vi "Mavlink CRC READ.vi"(11 "Byte IN":u8[](array[numeric])=[9, 19, 1, 1, 0, 0, 0, 0, 0, 2, 3, 81, 4, 3]) -> (3 "CRC":bool)   [LabVIEW 2023]
panel:
  out "Incoming Checksum":u16
  out "Calculated Checksum":u16
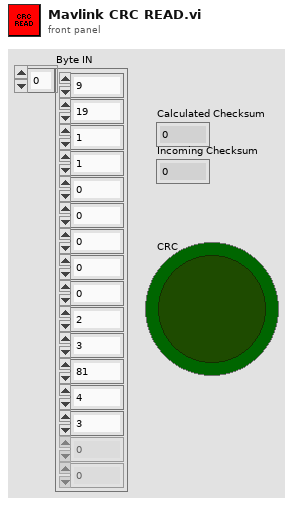
[diagram p1: front panel]
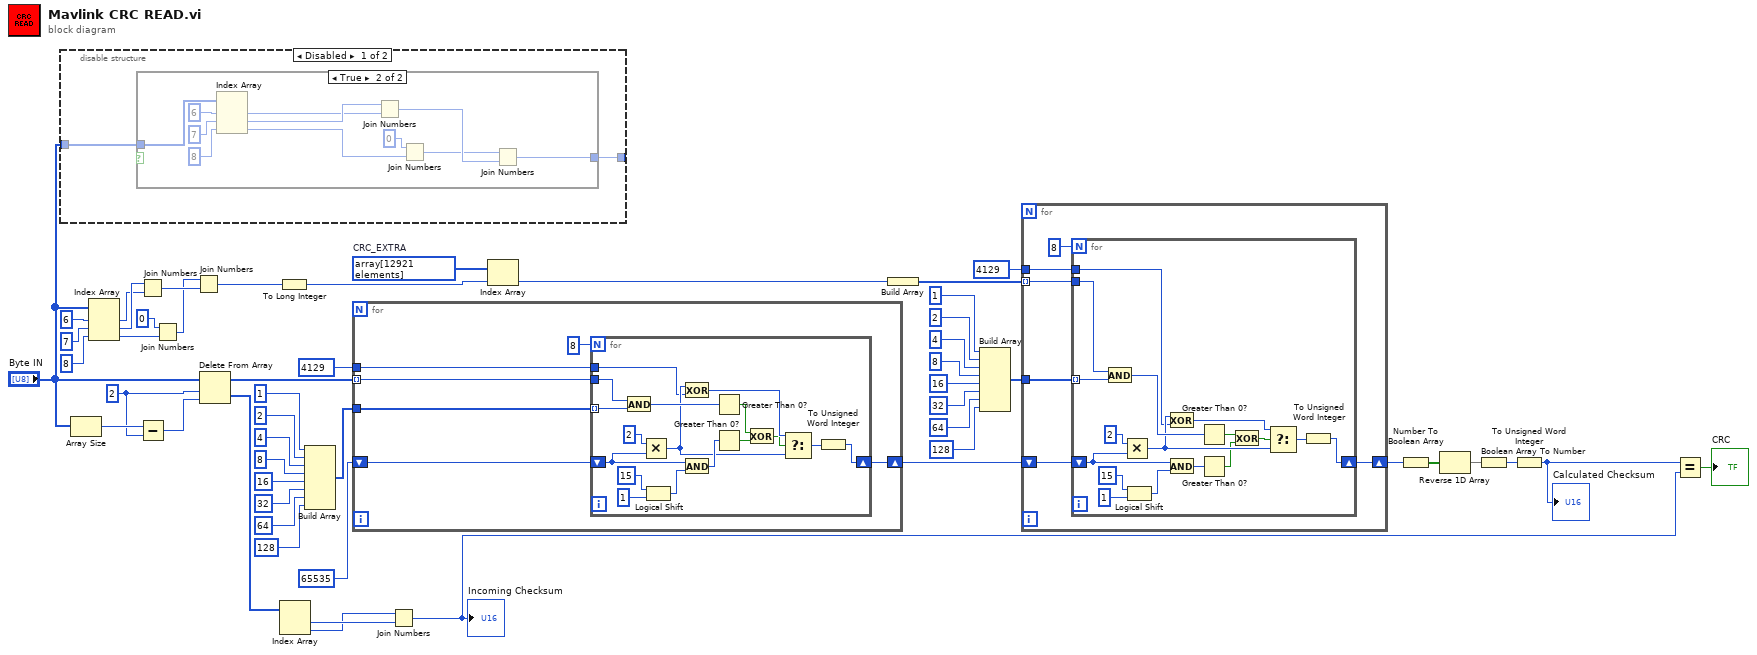
[diagram p0: block diagram]
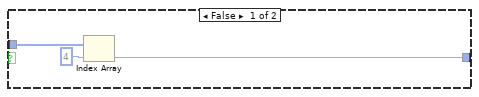
[diagram p2: hidden frame]
diagram:
  w20 = 2 ("y")
  w25 = u8[] array[12921 elements]  # CRC_EXTRA
  n1 = disable-structure shown="Disabled" {
    disable-tunnel: "Byte IN" -> [w53 _]
    disable-tunnel: [w52 _] -> _
    frame Disabled {
      n2 = case shown="True" {
        selector: _ -> [_ _]
        tunnel: w53 -> [w56 w57]
        tunnel: [w54 w58] -> w52
        frame False {
          n3 = Index Array(array=w56, index=4) -> (element=w54:u8)
        }
        frame True {
          n4 = Index Array(array=w57, index #1=6 ("index"), index #2=7 ("index"), index #3=8 ("index")) -> (element #1=w63:u8, element #2=w64:u8, element #3=w65:u8)
          n5 = Join Numbers(hi=w64, lo=w63) -> ((hi.lo)=w67:u16)
          n6 = Join Numbers(hi=u8 0, lo=w65) -> ((hi.lo)=w66:u16)
          n7 = Join Numbers(hi=w66, lo=w67) -> ((hi.lo)=w58:u32)
        }
      }
    }
    frame Enabled {
    }
  }
  n8 = Array Size(array="Byte IN") -> (size(s)=w22:i32)
  n9 = Index Array(array="Byte IN", index #1=6 ("index"), index #2=7 ("index"), index #3=8 ("index")) -> (element #1=w7:u8, element #2=w8:u8, element #3=w9:u8)
  n10 = Join Numbers(hi=w8, lo=w7) -> ((hi.lo)=w11:u16)
  n11 = Subtract(x=w22, y=w20) -> (x-y=w21:i32)
  n12 = Join Numbers(hi=u8 0, lo=w9) -> ((hi.lo)=w10:u16)
  n13 = Join Numbers(hi=w10, lo=w11) -> ((hi.lo)=w1:u32)
  n14 = Delete From Array(array="Byte IN", length=w20, index=w21) -> (deleted portion=w19:u8[], array with subset deleted=w18:u8[])
  n15 = To Long Integer(number=w1) -> (32bit integer=w12:i32)
  n16 = Index Array(array=w19) -> (element #1=w14:u8, element #2=w13:u8)  [unwired: 2 in]
  n17 = Build Array(u8 1, u8 2, u8 4, u8 8, u8 16, u8 32, u8 64, u8 128) -> (w42:u8[])
  n18 = for {
    shift-right: [w71] -> w26
    shift-left: u16 65535 -> [w73]
    tunnel: w18 -> [w70] mode=indexing
    tunnel: w42 -> [w69]
    tunnel: u16 4129 -> [w68]
    n19 = for {
      N: 8 -> [_]
      shift-right: [w89] -> w71
      shift-left: w73 -> [w79]
      tunnel: w69 -> [w80] mode=indexing
      tunnel: w70 -> [w75]
      tunnel: w68 -> [w74]
      n20 = And(x=w75, y=w80) -> (x .and. y?=w87:u8)
      n21 = Multiply(x=u16 2, y=w79) -> (x*y=w81:u16)
      n22 = Logical Shift(y=u16 15 ("Numeric"), x=u16 1 ("Numeric 2")) -> (x << y=w83:u16)
      n23 = Exclusive Or(1:w74, 2:w81) -> (0:w90:u16)
      n24 = And(x=w79, y=w83) -> (x .and. y?=w82:u16)
      n25 = Greater Than 0?(x=w87) -> (x > 0?=w86:bool)
      n26 = Greater Than 0?(x=w82) -> (x > 0?=w77:bool)
      n27 = Exclusive Or(1:w77, 2:w86) -> (0:w76:bool)
      n28 = Select(t=w90, s=w76, f=w81) -> (s? t:f=w88:u16)
      n29 = To Unsigned Word Integer(number=w88) -> (unsigned 16bit integer=w89:u16)
    }
  }
  n30 = Join Numbers(hi=w13, lo=w14) -> ((hi.lo)=w16:u16)
  "Incoming Checksum" <- w16
  n31 = Index Array(array=w25, index=w12) -> (element=w24:u8)
  n32 = Build Array(w24) -> (w23:u8[])
  n33 = Build Array(u8 1, u8 2, u8 4, u8 8, u8 16, u8 32, u8 64, u8 128) -> (w36:u8[])
  n34 = for {
    shift-right: [w94] -> w27
    shift-left: w26 -> [w96]
    tunnel: w36 -> [w93]
    tunnel: u16 4129 -> [w92]
    tunnel: w23 -> [w91] mode=indexing
    n35 = for {
      N: 8 -> [_]
      shift-right: [w112] -> w94
      shift-left: w96 -> [w102]
      tunnel: w93 -> [w103] mode=indexing
      tunnel: w91 -> [w98]
      tunnel: w92 -> [w97]
      n36 = And(x=w98, y=w103) -> (x .and. y?=w110:u8)
      n37 = Multiply(x=u16 2, y=w102) -> (x*y=w104:u16)
      n38 = Logical Shift(y=u16 15, x=u16 1) -> (x << y=w106:u16)
      n39 = Exclusive Or(1:w97, 2:w104) -> (0:w113:u16)
      n40 = And(x=w102, y=w106) -> (x .and. y?=w105:u16)
      n41 = Greater Than 0?(x=w110) -> (x > 0?=w109:bool)
      n42 = Greater Than 0?(x=w105) -> (x > 0?=w100:bool)
      n43 = Exclusive Or(1:w100, 2:w109) -> (0:w99:bool)
      n44 = Select(t=w113, s=w99, f=w104) -> (s? t:f=w111:u16)
      n45 = To Unsigned Word Integer(number=w111) -> (unsigned 16bit integer=w112:u16)
    }
  }
  n46 = Number To Boolean Array(number=w27) -> (Boolean array=w41:bool[])
  n47 = Reverse 1D Array(array=w41) -> (reversed array=w40:bool[])
  n48 = Boolean Array To Number(Boolean array=w40) -> (number=w39:u32)
  n49 = To Unsigned Word Integer(number=w39) -> (unsigned 16bit integer=w17:u16)
  "Calculated Checksum" <- w17
  n50 = Equal?(x=w17, y=w16) -> (x = y?=→"CRC":bool)
